vi "Generate Web Service Description.vi"(8 "error in (no error)":errorcluster, 11 "Description":T1) -> (0 "error out":errorcluster, 3 "Web Service Description String":string)   [LabVIEW 2020, in "Web Service Description.lvlib"]
uses:
  <vilib>/AppBuilder/Engine/WebServiceDescription/Web Service Description.lvlib
  <vilib>/AppBuilder/Engine/WebServiceDescription/XMLGen/XMLGen.lvlib
  <vilib>/AppBuilder/Engine/WebServiceDescription/LVDataTypes/LVType/LVType.lvclass
  <vilib>/AppBuilder/Engine/WebServiceDescription/Terminal Info.ctl
  <vilib>/AppBuilder/Engine/WebServiceDescription/Response.ctl
  <vilib>/AppBuilder/Engine/WebServiceDescription/URL Mapping Info.ctl
  <vilib>/AppBuilder/Engine/WebServiceDescription/Web Service Description Info.ctl
  <vilib>/AppBuilder/AB_Classes/Source/RESTfulVI/Configure_RESTfulVI/AB_RESTful_OutputFormat.ctl
  <vilib>/AppBuilder/AB_Classes/Source/RESTfulVI/Configure_RESTfulVI/AB_RESTful_OutputType.ctl
  <vilib>/AppBuilder/AB_Classes/RESTful/AB_RESTful_HTTPMethodType.ctl
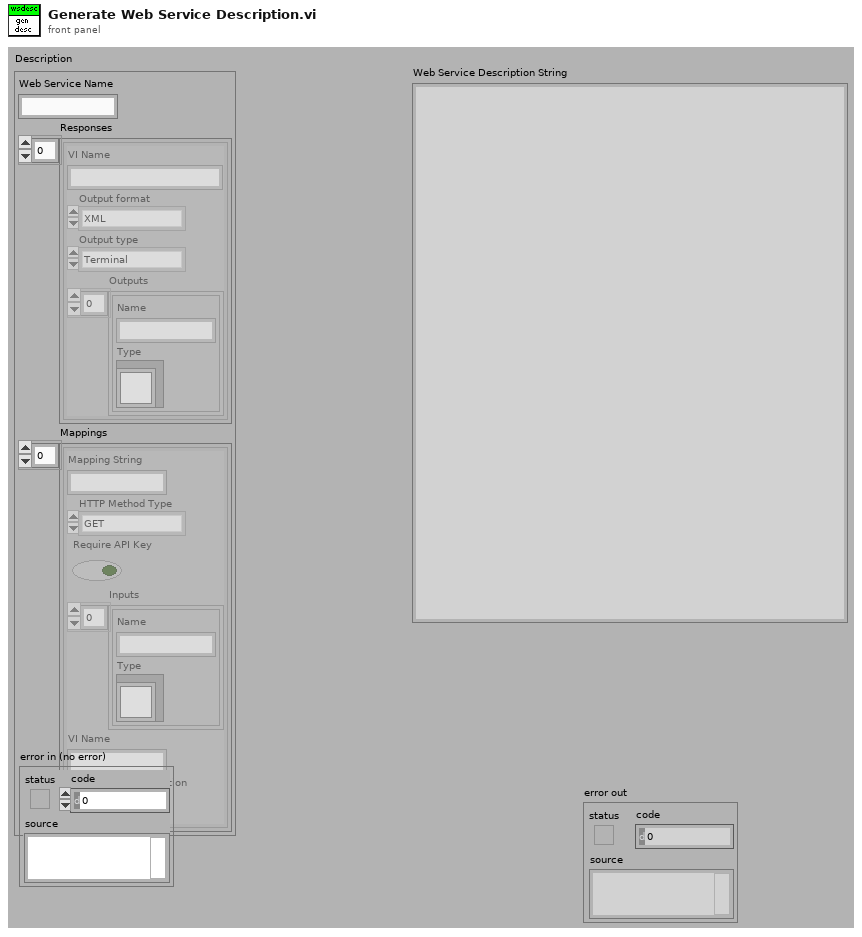
[diagram p1: front panel]
types:
  T1 = typedef "Web Service Description.lvlib/Web Service Description Info.ctl" = cluster{"Web Service Name":string, "Responses":T2[], "Mappings":T6[]}
  T2 = typedef "Web Service Description.lvlib/Response.ctl" = cluster{"VI Name":string, "Output format":T3, "Output type":T4, "Outputs":T5[]}
  T3 = typedef "AB_RESTful_OutputFormat.ctl" = enum32{"XML", "Text", "HTML", "JSON"}
  T4 = typedef "AB_RESTful_OutputType.ctl" = enum32{"Terminal", "Stream"}
  T5 = typedef "Web Service Description.lvlib/Terminal Info.ctl" = cluster{"Name":string, "Type":refnum<class "LVType.lvclass">}
  T6 = typedef "Web Service Description.lvlib/URL Mapping Info.ctl" = cluster{"Mapping String":string, "HTTP Method Type":T7, "Require API Key":bool, "Inputs":T5[], "VI Name":string, "Require Authentication":bool}
  T7 = typedef "AB_RESTful_HTTPMethodType.ctl" = enum32{"GET", "POST", "PUT", "DELETE"}
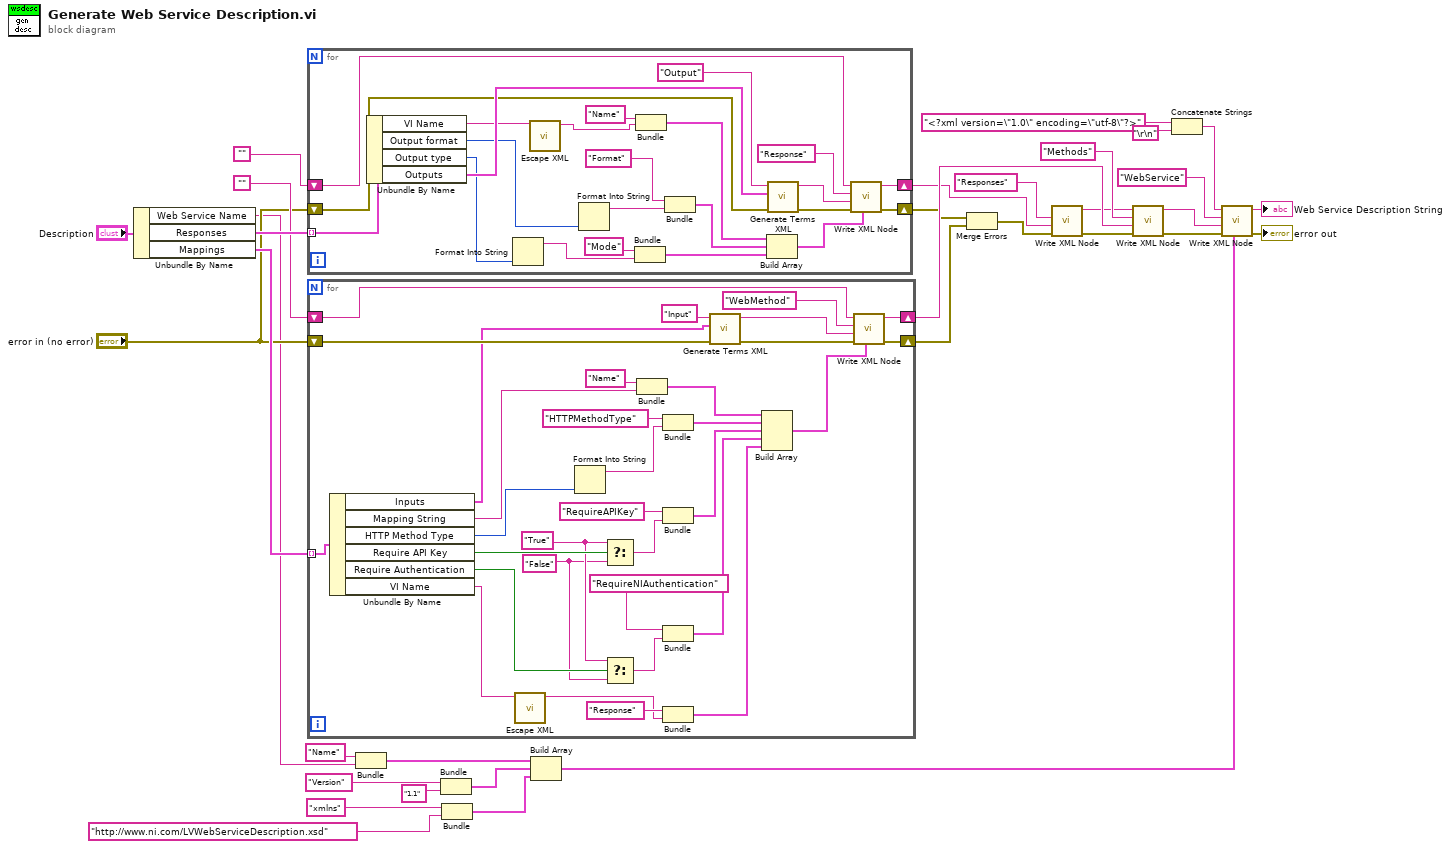
[diagram p0: block diagram]
diagram:
  n1 = Unbundle By Name("Description") -> ("Web Service Name"=w20:string, "Responses"=w32:T2[], "Mappings"=w30:T6[])
  n2 = for {
    tunnel: w32 -> [w56] mode=indexing
    shift-right: [w44] -> w24
    shift-left: "" -> [w45]
    shift-right: [w46] -> w15
    shift-left: "error in (no error)" -> [w49]
    n3 = Unbundle By Name(w56) -> ("VI Name"=w35:string, "Output format"=w40:T3, "Output type"=w38:T4, "Outputs"=w50:T5[])
    n4 = Format Into String(w38) -> (resulting string=w37:string)  [unwired: 3 in, 1 out]
    n5 = call <vilib>:"Escape XML.vi"("XML String In"=w35) -> ("XML String Out"=w34:string)  [unwired: 9 in, 1 out]
    n6 = Format Into String(w40) -> (resulting string=w39:string)  [unwired: 3 in, 1 out]
    n7 = Bundle("Mode", w37) -> (w36:cluster{string, string})  [unwired: 1 out]
    n8 = Bundle("Name", "XML String Out"=w34) -> (w52:cluster{string, "XML String Out":string})  [unwired: 1 out]
    n9 = Bundle("Format", w39) -> (w51:cluster{string, string})  [unwired: 1 out]
    n10 = Build Array(w52, w51, w36) -> (w48:cluster{string, "XML String Out":string}[])
    n11 = call <vilib>:"Generate Terms XML.vi"("error in (no error)"=w49, "Terminals"=w50, "Node Name"="Output" ("node")) -> ("error out"=w47:errorcluster, "XML out"=w42:string)  [unwired: 3 out]
    n12 = call <vilib>:"Write XML Node.vi"("attributes"=w48, "error in (no error)"=w47, "body"=w42, "node"="Response", "initial string"=w45) -> ("error out"=w46:errorcluster, "resulting string"=w44:string)  [unwired: 5 out]
  }
  n13 = for {
    tunnel: w30 -> [w88] mode=indexing
    shift-right: [w75] -> w27
    shift-left: "" -> [w76]
    shift-right: [w72] -> w14
    shift-left: "error in (no error)" -> [w70]
    w61 = "False"
    w62 = "True"
    n14 = Unbundle By Name(w88) -> ("Inputs"=w59:T5[], "Mapping String"=w83:string, "HTTP Method Type"=w67:T7, "Require API Key"=w82:bool, "Require Authentication"=w63:bool, "VI Name"=w58:string)
    n15 = call <vilib>:"Escape XML.vi"("XML String In"=w58) -> ("XML String Out"=w57:string)  [unwired: 9 in, 1 out]
    n16 = Format Into String(w67) -> (resulting string=w66:string)  [unwired: 3 in, 1 out]
    n17 = Select(t=w62, s=w82, f=w61) -> (s? t:f=w81:string)
    n18 = Select(t=w62, s=w63, f=w61) -> (s? t:f=w65:string)
    n19 = Bundle("Name", "Mapping String"=w83) -> (w80:cluster{string, "Mapping String":string})  [unwired: 1 out]
    n20 = Bundle("HTTPMethodType", w66) -> (w79:cluster{string, string})  [unwired: 1 out]
    n21 = Bundle("RequireAPIKey", w81) -> (w78:cluster{string, string})  [unwired: 1 out]
    n22 = Bundle("RequireNIAuthentication", w65) -> (w60:cluster{string, string})  [unwired: 1 out]
    n23 = Bundle("Response", "XML String Out"=w57) -> (w77:cluster{string, "XML String Out":string})  [unwired: 1 out]
    n24 = call <vilib>:"Generate Terms XML.vi"("error in (no error)"=w70, "Terminals"=w59, "Node Name"="Input" ("node")) -> ("error out"=w69:errorcluster, "XML out"=w68:string)  [unwired: 3 out]
    n25 = Build Array(w80, w79, w78, w60, w77) -> (w73:cluster{string, "XML String Out":string}[])
    n26 = call <vilib>:"Write XML Node.vi"("attributes"=w73, "error in (no error)"=w69, "body"=w68, "node"="WebMethod", "initial string"=w76) -> ("error out"=w72:errorcluster, "resulting string"=w75:string)  [unwired: 5 out]
  }
  n27 = Bundle("Name", "Web Service Name"=w20) -> (w19:cluster{string, "Web Service Name":string})  [unwired: 1 out]
  n28 = Bundle("Version", "1.1") -> (w18:cluster{string, string})  [unwired: 1 out]
  n29 = Bundle("xmlns", "http://www.ni.com/LVWebServiceDescription.xsd") -> (w1:cluster{string, string})  [unwired: 1 out]
  n30 = Build Array(w19, w18, w1) -> (w17:cluster{string, "Web Service Name":string}[])
  n31 = Merge Errors(w15, w14) -> (w13:errorcluster)
  n32 = call <vilib>:"Write XML Node.vi"("error in (no error)"=w13, "body"=w24, "node"="Responses") -> ("error out"=w16:errorcluster, "resulting string"=w11:string)  [unwired: 2 in, 5 out]
  n33 = call <vilib>:"Write XML Node.vi"("error in (no error)"=w16, "body"=w27, "node"="Methods", "initial string"=w11) -> ("error out"=w12:errorcluster, "resulting string"=w10:string)  [unwired: 1 in, 5 out]
  n34 = Concatenate Strings("<?xml version=\"1.0\" encoding=\"utf-8\"?>" ("string"), "\r\n") -> (w4:string)
  n35 = call <vilib>:"Write XML Node.vi"("attributes"=w17, "error in (no error)"=w12, "body"=w10, "node"="WebService", "initial string"=w4) -> ("error out"=→"error out":errorcluster, "resulting string"=→"Web Service Description String":string)  [unwired: 5 out]
